vi "dfd_Validate Quantizer.vi"(8 "error in (no error)":errorcluster, 10 "quantizer in":T1={"source"=0, "wl"=16, "iwl"=1, "overflow mode"=enum."Wrap", "rounding mode"=enum."Truncation", "signed?"=TRUE} {"source" items=["Coef a/k"=0, "Coef b/v"=7, "Input"=1, "Output"=2, "Multiplicand"=3, "Product"=4, "Sum"=5, "Delay"=6, "Gain"=8]}) -> (0 "error out":errorcluster, 1 "coef source?":bool, 2 "dup quantizer":T1={"source"=0, "wl"=16, "iwl"=1, "overflow mode"=enum."Wrap", "rounding mode"=enum."Truncation", "signed?"=TRUE} {"source" items=["Coef a/k"=0, "Coef b/v"=7, "Input"=1, "Output"=2, "Multiplicand"=3, "Product"=4, "Sum"=5, "Delay"=6, "Gain"=8]})   [LabVIEW 2017, in "NI_DigFilter_FXP.lvlib"]
uses:
  <vilib>/addons/Digital Filter Design/NI_DigFilter_FXP.lvlib
  <vilib>/addons/Digital Filter Design/_Objects.llb/dfd_Internal Quantization Settings.ctl
  <vilib>/addons/Digital Filter Design/_Objects.llb/dfd_Internal Quantization Srcs.ctl
  <vilib>/addons/Digital Filter Design/_Misc.llb/dfd_Error Handlers (Single).vi
  <vilib>/addons/Digital Filter Design/NI_DigFilterLicensed.lvlib
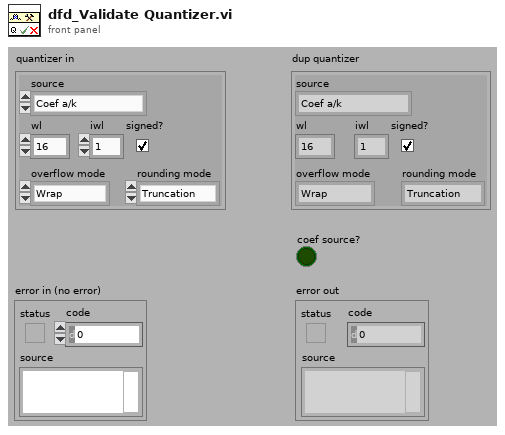
[diagram p1: front panel]
types:
  T1 = typedef "NI_DigFilterLicensed.lvlib/dfd_Internal Quantization Settings.ctl" = cluster{"source":T2, "wl":i16, "iwl":i16, "overflow mode":enum16{"Saturation", "Wrap"}, "rounding mode":enum16{"Nearest", "Truncation"}, "signed?":bool}
  T2 = typedef "NI_DigFilterLicensed.lvlib/dfd_Internal Quantization Srcs.ctl" = u16
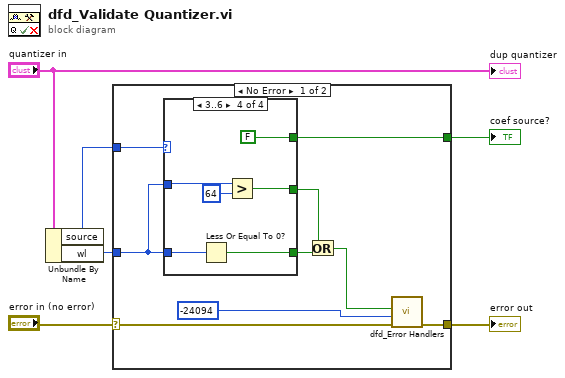
[diagram p0: block diagram]
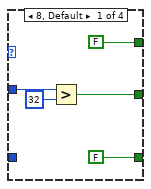
[diagram p2: hidden frame]
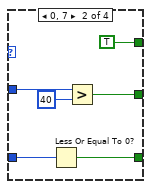
[diagram p3: hidden frame]
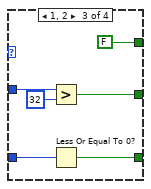
[diagram p4: hidden frame]
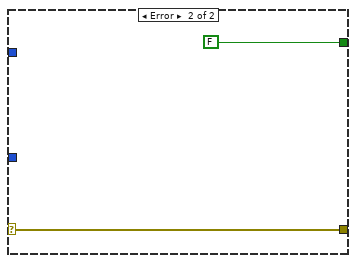
[diagram p5: hidden frame]
diagram:
  n1 = Unbundle By Name("quantizer in") -> ("source"=w2:T2, "wl"=w3:i16)
  n2 = case shown="No Error" "error in (no error)" {
    selector: "error in (no error)" -> [w14 w40]
    tunnel: [w13 w40] -> w4
    tunnel: w3 -> [w7 _]
    tunnel: w2 -> [w12 _]
    tunnel: [w11 FALSE] -> w1
    frame No Error {
      n3 = case shown="3..6" w12 {
        tunnel: [FALSE TRUE FALSE FALSE] -> w11
        tunnel: w7 -> [w19 w25 w31 w37]
        tunnel: [w17 w23 w29 w36] -> w10
        tunnel: [FALSE w21 w27 w34] -> w8
        tunnel: w7 -> [_ w22 w28 w35]
        frame 8, Default {
          n4 = Greater?(x=w19, y=i16 32) -> (0:w17:bool)
        }
        frame 0, 7 {
          n5 = Less Or Equal To 0?(x=w22) -> (x <= 0?=w21:bool)
          n6 = Greater?(x=w25, y=i16 40) -> (0:w23:bool)
        }
        frame 1, 2 {
          n7 = Greater?(x=w31, y=i16 32) -> (0:w29:bool)
          n8 = Less Or Equal To 0?(x=w28) -> (x <= 0?=w27:bool)
        }
        frame 3..6 {
          n9 = Less Or Equal To 0?(x=w35) -> (x <= 0?=w34:bool)
          n10 = Greater?(x=w37, y=i16 64) -> (0:w36:bool)
        }
      }
      n11 = Or(x=w10, y=w8) -> (x .or. y?=w9:bool)
      n12 = call-poly <vilib>:"dfd_Error Handlers.vi"("error in (no error)"=w14, "error code"=-24094 ("ERR_INVALID_WL"), "condition failed?"=w9) -> ("error out"=w13:errorcluster)  [unwired: 8 out]
    }
    frame Error {
    }
  }
  "error out" <- w4
  "coef source?" <- w1
  "dup quantizer" <- "quantizer in"
